vi "call_DLL.vi"() -> ()   [LabVIEW 2013]
uses:
  CircularArea/CircularArea.lvlib
  CircularArea.dll
panel:
  out "Numeric 2":dbl
  in  "Numeric":dbl
  out "output area":dbl
  in  "input radius":dbl
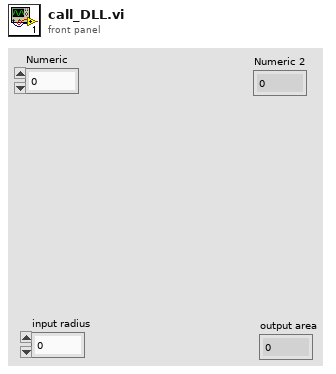
[diagram p1: front panel]
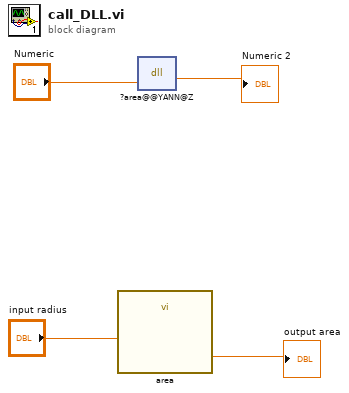
[diagram p0: block diagram]
diagram:
  n1 = call "area.vi"("radius"="input radius") -> ("function return"=→"output area":dbl)  [unwired: 10 in]
  n2 = dll-call lib="D:/congxin/labview/CircularArea.dll" fn="?area@@YANN@Z"("radius"="Numeric") -> ("return type"=→"Numeric 2":dbl)  [unwired: 4 in, 2 out]
